vi "c_buf.vi"(2 "Numeric 2":i32, 3 "Array":string[](array[string]), 4 "Query":string) -> (0 "Numeric":i32, 1 "Array 2":string[](array[string]))   [LabVIEW 2010]
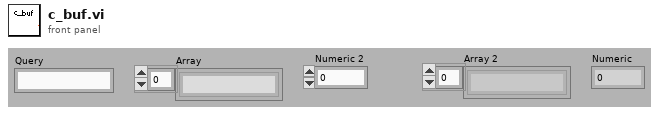
[diagram p1: front panel]
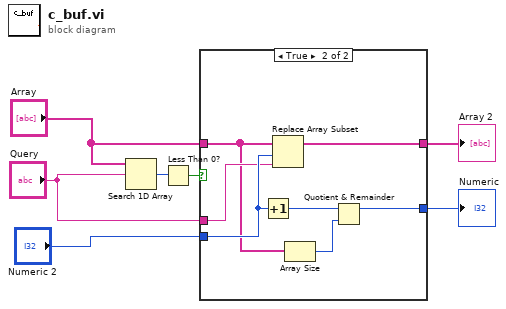
[diagram p0: block diagram]
diagram:
  n1 = Search 1D Array(1D array="Array", element="Query") -> (index of element=w7:i32)  [unwired: 1 in]
  n2 = Less Than 0?(x=w7) -> (x < 0?=w6:bool)
  n3 = case shown="True" w6 {
    tunnel: "Array" -> [w9 w10]
    tunnel: "Numeric 2" -> [w8 w15]
    tunnel: [w8 w14] -> w3
    tunnel: [w9 w13] -> w2
    tunnel: "Query" -> [_ w11]
    frame False {
    }
    frame True {
      n4 = Increment(x=w15) -> (x+1=w16:i32)
      n5 = Replace Array Subset(array=w10, new element=w11, index=w15) -> (w13:string[])
      n6 = Array Size(array=w10) -> (size(s)=w12:i32)
      n7 = Quotient & Remainder(x=w16, y=w12) -> (x-y*floor(x/y)=w14:i32)  [unwired: 1 out]
    }
  }
  "Numeric" <- w3
  "Array 2" <- w2
